vi "Ctor.vi"(8 "error in (no error)":errorcluster, 11 "BluePlotHandle in":refnum<class "RocketPlotHandle.lvclass">) -> (0 "error out":errorcluster, 3 "BluePlotHandle out":refnum<class "RocketPlotHandle.lvclass">)   [LabVIEW 2021, in "RocketPlotHandle.lvclass"]
uses:
  RocketPlotHandle.lvclass
  TypeDefs/plot handle queue data.ctl
  TypeDefs/Plot QSM action.ctl
  RocketPlotHandle.lvclass/RocketPlotHandle.ctl
  RocketPlot.lvlib
  SubVIs/callback type.ctl
  SubVIs/callback data.ctl
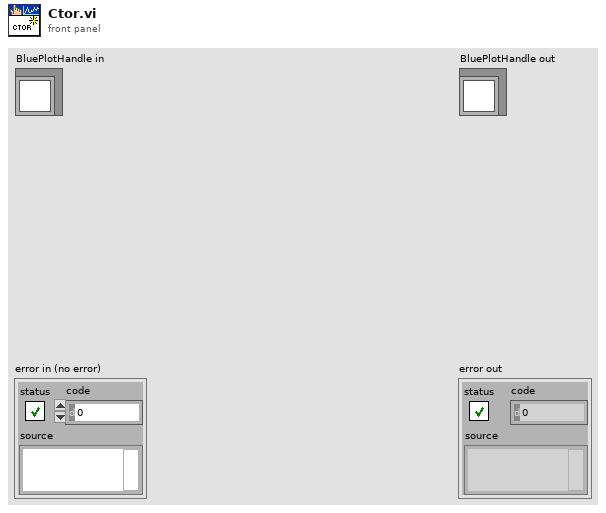
[diagram p1: front panel]
types:
  T1 = typedef "RocketPlotHandle.lvclass/callback data.ctl" = cluster{"Type":T2, "data":variant, "owning subpanel":refnum<vi>}
  T2 = typedef "RocketPlotHandle.lvclass/callback type.ctl" = enum16{"Maximize", "ShortcutMenu"}
  T3 = typedef "RocketPlot.lvlib/plot handle queue data.ctl" = cluster{"action":T4, "data":variant}
  T4 = typedef "RocketPlot.lvlib/Plot QSM action.ctl" = enum16{"Get Config", "Load Config", "Set TimeToPlot", "Clear Config"}
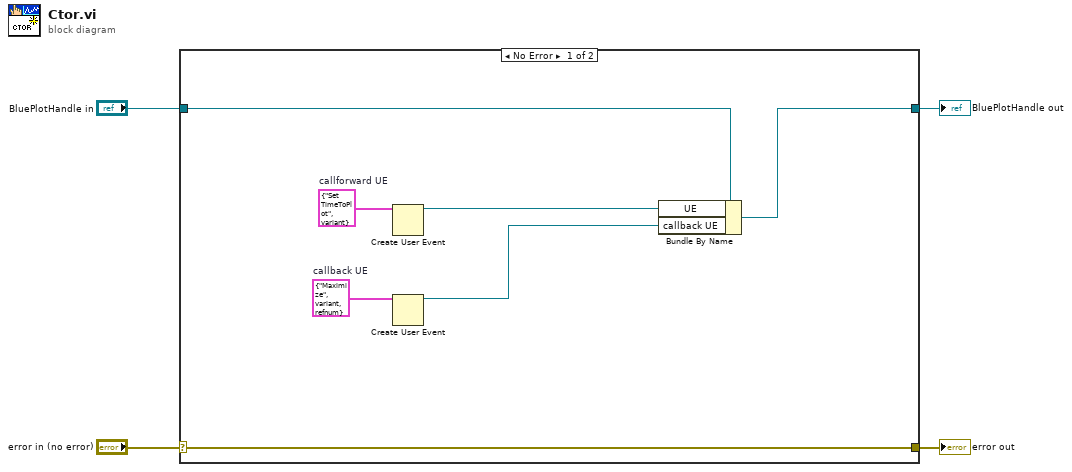
[diagram p0: block diagram]
diagram:
  n1 = case shown="No Error" "error in (no error)" {
    selector: "error in (no error)" -> [w11 w13]
    tunnel: [w11 w13] -> w3
    tunnel: [w7 w12] -> w1
    tunnel: "BluePlotHandle in" -> [w9 w12]
    frame No Error {
      w6 = T1 {"Type"=enum."Maximize", "data"=variant, "owning subpanel"=refnum}  # callback UE
      w10 = T3 {"action"=enum."Set TimeToPlot", "data"=variant}  # callforward UE
      n2 = Create User Event(user event datatype=w10) -> (user event=w8:refnum<user-event>)  [unwired: 1 in, 1 out]
      n3 = Create User Event(user event datatype=w6) -> (user event=w5:refnum<user-event>)  [unwired: 1 in, 1 out]
      n4 = Bundle By Name(cluster=w9, "UE"=w8, "callback UE"=w5) -> (w7:refnum<class "RocketPlotHandle.lvclass">)
    }
    frame Error {
    }
  }
  "error out" <- w3
  "BluePlotHandle out" <- w1
